vi "Data_Acquisition_10 sensors.vi"() -> ()   [LabVIEW 2020]
uses:
  <vilib>/Instr/_visa.llb/VISA Configure Serial Port (Instr).vi
panel:
  out "Path S10":path
  out "Path S9":path
  out "Path S8":path
  out "Path S7":path
  out "Path S6":path
  out "Path S5":path
  out "Path S3":path
  out "Path S4":path
  out "Path S2":path
  out "Path S1":path
  in  "Trial Select":string(combo)
  in  "Person Select":string(combo)
  in  "Gesture Select":string(combo)
  out "Myoware 2":dbl[](array[numeric]) format="%#.11g"
  out "FSR 8":dbl[](array[numeric]) format="%#.11g"
  out "FSR 7":dbl[](array[numeric]) format="%#.11g"
  out "FSR 6":dbl[](array[numeric]) format="%#.11g"
  out "FSR 5":dbl[](array[numeric]) format="%#.11g"
  out "Myoware 1":dbl[](array[numeric]) format="%#.11g"
  out "FSR 4":dbl[](array[numeric]) format="%#.11g"
  out "FSR 3":dbl[](array[numeric]) format="%#.11g"
  out "Myoware 2 Chart":dbl[](graph)
  out "FSR 8 Chart":dbl[](graph)
  out "FSR 7 Chart":dbl[](graph)
  out "FSR 6 Chart":dbl[](graph)
  out "FSR 5 Chart":dbl[](graph)
  out "Myoware 1 Chart":dbl[](graph)
  out "FSR 4 Chart":dbl[](graph)
  out "FSR 3 Chart":dbl[](graph)
  out "FSR 2 Chart":dbl[](graph)
  out "FSR 1 Chart":dbl[](graph)
  out "FSR 2":dbl[](array[numeric]) format="%#.11g"
  out "FSR 1":dbl[](array[numeric]) format="%#.11g"
  in  "COM Port Select":refnum<visa-resource-name>
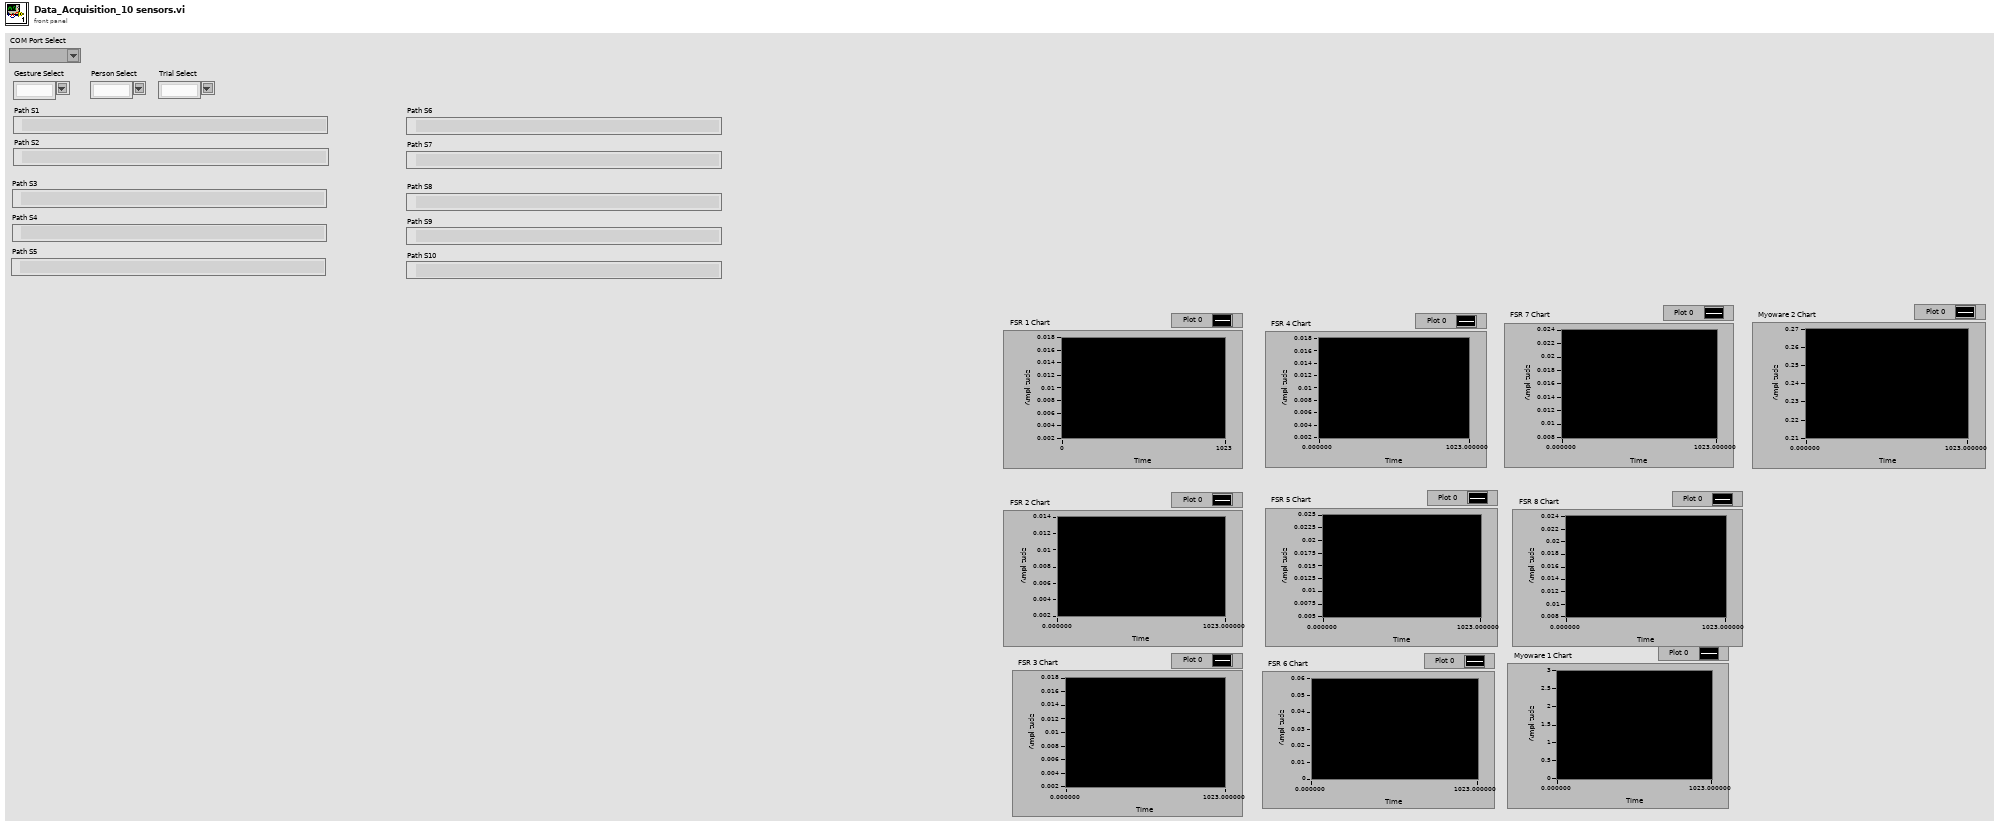
[diagram p1: front panel]
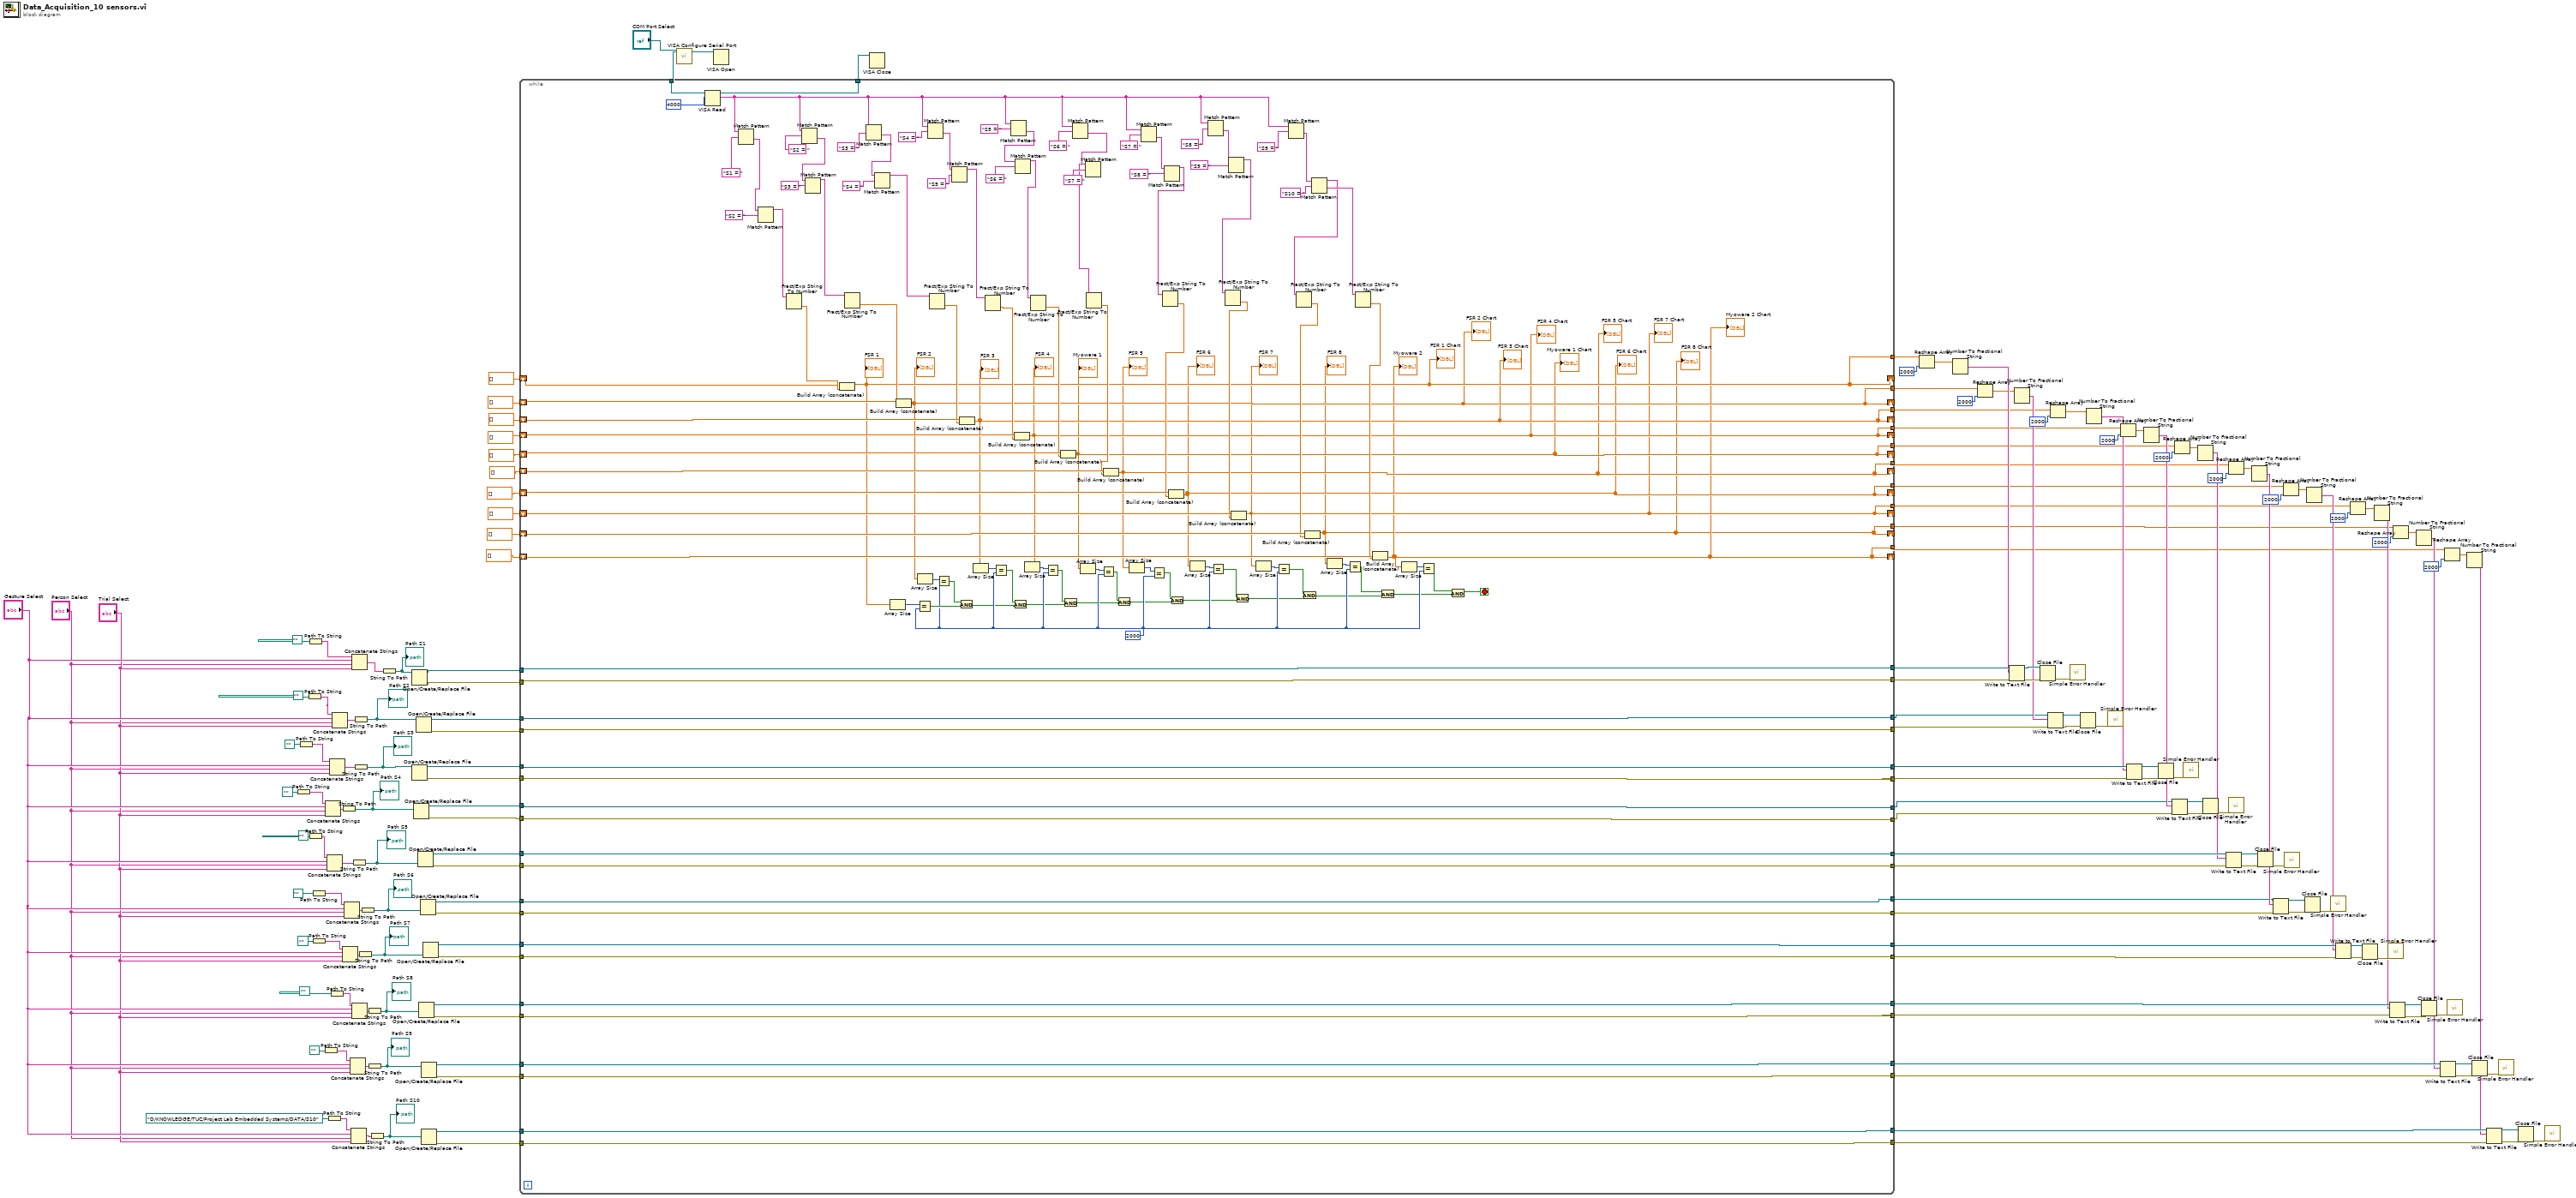
[diagram p0: block diagram]
diagram:
  n1 = Path To String(path=path "" ("file path (use dialog)")) -> (string=w142:string)
  n2 = Path To String(path=path "" ("file path (use dialog)")) -> (string=w139:string)
  n3 = Path To String(path=path "" ("file path (use dialog)")) -> (string=w146:string)
  n4 = Path To String(path=path "" ("file path (use dialog)")) -> (string=w152:string)
  n5 = Path To String(path=path "" ("file path (use dialog)")) -> (string=w136:string)
  n6 = Path To String(path=path "" ("file path (use dialog)")) -> (string=w130:string)
  n7 = Path To String(path=path "" ("file path (use dialog)")) -> (string=w133:string)
  n8 = Path To String(path=path "" ("file path (use dialog)")) -> (string=w124:string)
  n9 = Concatenate Strings(w142, "Gesture Select", "Person Select", "Trial Select") -> (w144:string)
  n10 = Path To String(path=path "D:/KNOWLEDGE/TUC/Project Lab Embedded Systems/DATA/S10" ("file path (use dialog)")) -> (string=w122:string)
  n11 = Concatenate Strings(w136, "Gesture Select", "Person Select", "Trial Select") -> (w138:string)
  n12 = Concatenate Strings(w139, "Gesture Select", "Person Select", "Trial Select") -> (w141:string)
  n13 = Path To String(path=path "" ("file path (use dialog)")) -> (string=w127:string)
  n14 = Concatenate Strings(w146, "Gesture Select", "Person Select", "Trial Select") -> (w145:string)
  n15 = String To Path(string=w144) -> (path=w96:path)
  "Path S4" <- w96
  n16 = Concatenate Strings(w130, "Gesture Select", "Person Select", "Trial Select") -> (w132:string)
  n17 = Concatenate Strings(w133, "Gesture Select", "Person Select", "Trial Select") -> (w135:string)
  n18 = Concatenate Strings(w124, "Gesture Select", "Person Select", "Trial Select") -> (w126:string)
  n19 = Concatenate Strings(w122, "Gesture Select", "Person Select", "Trial Select") -> (w123:string)
  n20 = Concatenate Strings(w152, "Gesture Select", "Person Select", "Trial Select") -> (w151:string)
  n21 = String To Path(string=w138) -> (path=w99:path)
  "Path S5" <- w99
  n22 = Concatenate Strings(w127, "Gesture Select", "Person Select", "Trial Select") -> (w129:string)
  n23 = String To Path(string=w145) -> (path=w91:path)
  "Path S2" <- w91
  n24 = String To Path(string=w141) -> (path=w97:path)
  "Path S3" <- w97
  n25 = String To Path(string=w132) -> (path=w92:path)
  "Path S7" <- w92
  n26 = String To Path(string=w135) -> (path=w98:path)
  "Path S6" <- w98
  n27 = String To Path(string=w126) -> (path=w94:path)
  "Path S9" <- w94
  n28 = String To Path(string=w129) -> (path=w93:path)
  "Path S8" <- w93
  n29 = String To Path(string=w123) -> (path=w95:path)
  "Path S10" <- w95
  n30 = String To Path(string=w151) -> (path=w148:path)
  "Path S1" <- w148
  n31 = Open/Create/Replace File(file path (use dialog)=w148) -> (refnum out=w150:refnum<file>, error out=w149:errorcluster)  [unwired: 5 in, 1 out]
  n32 = Open/Create/Replace File(file path (use dialog)=w97) -> (refnum out=w115:refnum<file>, error out=w114:errorcluster)  [unwired: 5 in, 1 out]
  n33 = Open/Create/Replace File(file path (use dialog)=w96) -> (refnum out=w113:refnum<file>, error out=w112:errorcluster)  [unwired: 5 in, 1 out]
  n34 = Open/Create/Replace File(file path (use dialog)=w91) -> (refnum out=w117:refnum<file>, error out=w116:errorcluster)  [unwired: 5 in, 1 out]
  n35 = Open/Create/Replace File(file path (use dialog)=w99) -> (refnum out=w111:refnum<file>, error out=w110:errorcluster)  [unwired: 5 in, 1 out]
  n36 = Open/Create/Replace File(file path (use dialog)=w93) -> (refnum out=w104:refnum<file>, error out=w105:errorcluster)  [unwired: 5 in, 1 out]
  n37 = Open/Create/Replace File(file path (use dialog)=w98) -> (refnum out=w108:refnum<file>, error out=w109:errorcluster)  [unwired: 5 in, 1 out]
  n38 = Open/Create/Replace File(file path (use dialog)=w94) -> (refnum out=w102:refnum<file>, error out=w103:errorcluster)  [unwired: 5 in, 1 out]
  n39 = Open/Create/Replace File(file path (use dialog)=w95) -> (refnum out=w100:refnum<file>, error out=w101:errorcluster)  [unwired: 5 in, 1 out]
  n40 = Open/Create/Replace File(file path (use dialog)=w92) -> (refnum out=w106:refnum<file>, error out=w107:errorcluster)  [unwired: 5 in, 1 out]
  n41 = call-poly "VISA Configure Serial Port"("VISA resource name"="COM Port Select") -> ("VISA resource name out"=w166:refnum<visa-resource-name>)  [unwired: 13 in, 1 out]
  n42 = VISA Open(VISA resource name=w166) -> (VISA resource name=w155:refnum<visa-resource-name>)  [unwired: 4 in, 1 out]
  n43 = while {
    shift-right: [w195] -> _
    shift-left: dbl[] [] -> [w288]
    shift-right: [w198] -> _
    shift-left: dbl[] [] -> [w199]
    shift-right: [w192] -> _
    shift-left: dbl[] [] -> [w283]
    shift-right: [w189] -> _
    shift-left: dbl[] [] -> [w279]
    shift-right: [w186] -> _
    shift-left: dbl[] [] -> [w278]
    shift-right: [w185] -> _
    shift-left: dbl[] [] -> [w282]
    shift-right: [w184] -> _
    shift-left: dbl[] [] -> [w277]
    shift-right: [w183] -> _
    shift-left: dbl[] [] -> [w281]
    shift-right: [w174] -> _
    shift-left: dbl[] [] -> [w280]
    shift-right: [w182] -> _
    shift-left: dbl[] [] -> [w276]
    tunnel: w155 -> [w239]
    tunnel: [w229] -> w154
    tunnel: w150 -> [w197]
    tunnel: w149 -> [w196]
    tunnel: w117 -> [w194]
    tunnel: w116 -> [w193]
    tunnel: [w193] -> w73
    tunnel: [w194] -> w74
    tunnel: w115 -> [w191]
    tunnel: w114 -> [w190]
    tunnel: w113 -> [w188]
    tunnel: w112 -> [w187]
    tunnel: w111 -> [w171]
    tunnel: w110 -> [w170]
    tunnel: w109 -> [w172]
    tunnel: w108 -> [w173]
    tunnel: w107 -> [w175]
    tunnel: w106 -> [w169]
    tunnel: w105 -> [w177]
    tunnel: w104 -> [w176]
    tunnel: w103 -> [w179]
    tunnel: w102 -> [w178]
    tunnel: w101 -> [w181]
    tunnel: w100 -> [w180]
    tunnel: [w191] -> w68
    tunnel: [w190] -> w67
    tunnel: [w188] -> w56
    tunnel: [w187] -> w55
    tunnel: [w171] -> w51
    tunnel: [w170] -> w50
    tunnel: [w173] -> w38
    tunnel: [w172] -> w37
    tunnel: [w169] -> w33
    tunnel: [w175] -> w32
    tunnel: [w176] -> w28
    tunnel: [w177] -> w27
    tunnel: [w178] -> w23
    tunnel: [w179] -> w22
    tunnel: [w180] -> w18
    tunnel: [w181] -> w17
    tunnel: [w198] -> w89
    tunnel: [w197] -> w84
    tunnel: [w196] -> w83
    tunnel: [w195] -> w76
    tunnel: [w192] -> w70
    tunnel: [w189] -> w61
    tunnel: [w186] -> w47
    tunnel: [w185] -> w43
    tunnel: [w184] -> w14
    tunnel: [w183] -> w10
    tunnel: [w174] -> w6
    tunnel: [w182] -> w2
    stop <- w168 stop-if-true
    w267 = 2000 ("y")
    n44 = VISA Read(VISA resource name=w239, byte count=u32 4000) -> (VISA resource name out=w229:refnum<visa-resource-name>, read buffer=w204:string)  [unwired: 1 in, 2 out]
    n45 = Match Pattern(string=w204, regular expression="S1 = ") -> (after substring=w225:string)  [unwired: 1 in, 3 out]
    n46 = Match Pattern(string=w225, regular expression="S2 = ") -> (before substring=w226:string)  [unwired: 1 in, 3 out]
    n47 = Fract/Exp String To Number(string=w226) -> (number=w230:dbl)  [unwired: 3 in, 1 out]
    n48 = Match Pattern(string=w204, regular expression="S2 = ") -> (after substring=w223:string)  [unwired: 1 in, 3 out]
    n49 = Match Pattern(string=w223, regular expression="S3 = ") -> (before substring=w222:string)  [unwired: 1 in, 3 out]
    n50 = Build Array (concatenate)(w199, w230) -> (w198:dbl[])
    "FSR 1" <- w198
    "FSR 1 Chart" <- w198
    n51 = Fract/Exp String To Number(string=w222) -> (number=w231:dbl)  [unwired: 3 in, 1 out]
    n52 = Match Pattern(string=w204, regular expression="S3 = ") -> (after substring=w220:string)  [unwired: 1 in, 3 out]
    n53 = Match Pattern(string=w220, regular expression="S4 = ") -> (before substring=w219:string)  [unwired: 1 in, 3 out]
    n54 = Array Size(array=w198) -> (size(s)=w286:i32)
    n55 = Build Array (concatenate)(w288, w231) -> (w195:dbl[])
    "FSR 2" <- w195
    "FSR 2 Chart" <- w195
    n56 = Array Size(array=w195) -> (size(s)=w287:i32)
    n57 = Equal?(x=w286, y=w267) -> (x = y?=w284:bool)
    n58 = Match Pattern(string=w204, regular expression="S4 = ") -> (after substring=w217:string)  [unwired: 1 in, 3 out]
    n59 = Fract/Exp String To Number(string=w219) -> (number=w232:dbl)  [unwired: 3 in, 1 out]
    n60 = Equal?(x=w287, y=w267) -> (x = y?=w285:bool)
    n61 = Match Pattern(string=w217, regular expression="S5 = ") -> (before substring=w216:string)  [unwired: 1 in, 3 out]
    n62 = And(x=w285, y=w284) -> (x .and. y?=w265:bool)
    n63 = Build Array (concatenate)(w283, w232) -> (w192:dbl[])
    "FSR 3 Chart" <- w192
    "FSR 3" <- w192
    n64 = Array Size(array=w192) -> (size(s)=w275:i32)
    n65 = Fract/Exp String To Number(string=w216) -> (number=w233:dbl)  [unwired: 3 in, 1 out]
    n66 = Equal?(x=w275, y=w267) -> (x = y?=w266:bool)
    n67 = Match Pattern(string=w204, regular expression="S5 = ") -> (after substring=w214:string)  [unwired: 1 in, 3 out]
    n68 = And(x=w266, y=w265) -> (x .and. y?=w264:bool)
    n69 = Build Array (concatenate)(w279, w233) -> (w189:dbl[])
    "FSR 4 Chart" <- w189
    "FSR 4" <- w189
    n70 = Match Pattern(string=w214, regular expression="S6 = ") -> (before substring=w213:string)  [unwired: 1 in, 3 out]
    n71 = Array Size(array=w189) -> (size(s)=w274:i32)
    n72 = Fract/Exp String To Number(string=w213) -> (number=w234:dbl)  [unwired: 3 in, 1 out]
    n73 = Equal?(x=w274, y=w267) -> (x = y?=w263:bool)
    n74 = Build Array (concatenate)(w278, w234) -> (w186:dbl[])
    "Myoware 1 Chart" <- w186
    "Myoware 1" <- w186
    n75 = And(x=w263, y=w264) -> (x .and. y?=w262:bool)
    n76 = Match Pattern(string=w204, regular expression="S6 = ") -> (after substring=w211:string)  [unwired: 1 in, 3 out]
    n77 = Array Size(array=w186) -> (size(s)=w273:i32)
    n78 = Match Pattern(string=w211, regular expression="S7 = ") -> (before substring=w210:string)  [unwired: 1 in, 3 out]
    n79 = Fract/Exp String To Number(string=w210) -> (number=w235:dbl)  [unwired: 3 in, 1 out]
    n80 = Equal?(x=w273, y=w267) -> (x = y?=w261:bool)
    n81 = Build Array (concatenate)(w282, w235) -> (w185:dbl[])
    "FSR 5 Chart" <- w185
    "FSR 5" <- w185
    n82 = And(x=w261, y=w262) -> (x .and. y?=w260:bool)
    n83 = Array Size(array=w185) -> (size(s)=w272:i32)
    n84 = Match Pattern(string=w204, regular expression="S7 = ") -> (after substring=w200:string)  [unwired: 1 in, 3 out]
    n85 = Equal?(x=w272, y=w267) -> (x = y?=w259:bool)
    n86 = Match Pattern(string=w200, regular expression="S8 = ") -> (before substring=w208:string)  [unwired: 1 in, 3 out]
    n87 = Fract/Exp String To Number(string=w208) -> (number=w236:dbl)  [unwired: 3 in, 1 out]
    n88 = Build Array (concatenate)(w277, w236) -> (w184:dbl[])
    "FSR 6 Chart" <- w184
    "FSR 6" <- w184
    n89 = And(x=w259, y=w260) -> (x .and. y?=w258:bool)
    n90 = Array Size(array=w184) -> (size(s)=w271:i32)
    n91 = Match Pattern(string=w204, regular expression="S8 = ") -> (after substring=w206:string)  [unwired: 1 in, 3 out]
    n92 = Equal?(x=w271, y=w267) -> (x = y?=w257:bool)
    n93 = Match Pattern(string=w206, regular expression="S9 = ") -> (before substring=w205:string)  [unwired: 1 in, 3 out]
    n94 = Fract/Exp String To Number(string=w205) -> (number=w237:dbl)  [unwired: 3 in, 1 out]
    n95 = Build Array (concatenate)(w281, w237) -> (w183:dbl[])
    "FSR 7 Chart" <- w183
    "FSR 7" <- w183
    n96 = And(x=w257, y=w258) -> (x .and. y?=w256:bool)
    n97 = Array Size(array=w183) -> (size(s)=w270:i32)
    n98 = Equal?(x=w270, y=w267) -> (x = y?=w255:bool)
    n99 = Match Pattern(string=w204, regular expression="S9 = ") -> (after substring=w202:string)  [unwired: 1 in, 3 out]
    n100 = And(x=w255, y=w256) -> (x .and. y?=w254:bool)
    n101 = Match Pattern(string=w202, regular expression="S10 = ") -> (before substring=w249:string, after substring=w250:string)  [unwired: 1 in, 2 out]
    n102 = Fract/Exp String To Number(string=w249) -> (number=w238:dbl)  [unwired: 3 in, 1 out]
    n103 = Build Array (concatenate)(w280, w238) -> (w174:dbl[])
    "FSR 8 Chart" <- w174
    "FSR 8" <- w174
    n104 = Array Size(array=w174) -> (size(s)=w269:i32)
    n105 = Equal?(x=w269, y=w267) -> (x = y?=w253:bool)
    n106 = Fract/Exp String To Number(string=w250) -> (number=w201:dbl)  [unwired: 3 in, 1 out]
    n107 = Build Array (concatenate)(w276, w201) -> (w182:dbl[])
    "Myoware 2 Chart" <- w182
    "Myoware 2" <- w182
    n108 = And(x=w253, y=w254) -> (x .and. y?=w252:bool)
    n109 = Array Size(array=w182) -> (size(s)=w268:i32)
    n110 = Equal?(x=w268, y=w267) -> (x = y?=w251:bool)
    n111 = And(x=w251, y=w252) -> (x .and. y?=w168:bool)
  }
  n112 = VISA Close(VISA resource name=w154) -> ()  [unwired: 1 in, 1 out]
  n113 = Reshape Array(w89, 2000 ("dimension size")) -> (w88:dbl[])
  n114 = Number To Fractional String(number=w88) -> (F-format string=w82:string[])  [unwired: 3 in]
  n115 = Reshape Array(w76, 2000 ("dimension size")) -> (w77:dbl[])
  n116 = Write to Text File(file (use dialog)=w84, text=w82, error in=w83) -> (refnum out=w86:refnum<file>, error out=w85:errorcluster)  [unwired: 1 in, 1 out]
  n117 = Number To Fractional String(number=w77) -> (F-format string=w75:string[])  [unwired: 3 in]
  n118 = Close File(refnum=w86, error in=w85) -> (error out=w87:errorcluster)  [unwired: 1 out]
  n119 = Write to Text File(file (use dialog)=w74, text=w75, error in=w73) -> (refnum out=w80:refnum<file>, error out=w79:errorcluster)  [unwired: 1 in, 1 out]
  n120 = Reshape Array(w70, 2000 ("dimension size")) -> (w71:dbl[])
  n121 = call <vilib>:"Simple Error Handler.vi"("error in (no error)"=w87) -> ()  [unwired: 4 in, 5 out]
  n122 = Close File(refnum=w80, error in=w79) -> (error out=w81:errorcluster)  [unwired: 1 out]
  n123 = Number To Fractional String(number=w71) -> (F-format string=w64:string[])  [unwired: 3 in]
  n124 = call <vilib>:"Simple Error Handler.vi"("error in (no error)"=w81) -> ()  [unwired: 4 in, 5 out]
  n125 = Reshape Array(w61, 2000 ("dimension size")) -> (w62:dbl[])
  n126 = Write to Text File(file (use dialog)=w68, text=w64, error in=w67) -> (refnum out=w66:refnum<file>, error out=w65:errorcluster)  [unwired: 1 in, 1 out]
  n127 = Number To Fractional String(number=w62) -> (F-format string=w57:string[])  [unwired: 3 in]
  n128 = Close File(refnum=w66, error in=w65) -> (error out=w69:errorcluster)  [unwired: 1 out]
  n129 = Write to Text File(file (use dialog)=w56, text=w57, error in=w55) -> (refnum out=w59:refnum<file>, error out=w58:errorcluster)  [unwired: 1 in, 1 out]
  n130 = Reshape Array(w47, 2000 ("dimension size")) -> (w48:dbl[])
  n131 = call <vilib>:"Simple Error Handler.vi"("error in (no error)"=w69) -> ()  [unwired: 4 in, 5 out]
  n132 = Number To Fractional String(number=w48) -> (F-format string=w46:string[])  [unwired: 3 in]
  n133 = Close File(refnum=w59, error in=w58) -> (error out=w60:errorcluster)  [unwired: 1 out]
  n134 = Write to Text File(file (use dialog)=w51, text=w46, error in=w50) -> (refnum out=w53:refnum<file>, error out=w52:errorcluster)  [unwired: 1 in, 1 out]
  n135 = Reshape Array(w43, 2000 ("dimension size")) -> (w44:dbl[])
  n136 = call <vilib>:"Simple Error Handler.vi"("error in (no error)"=w60) -> ()  [unwired: 4 in, 5 out]
  n137 = Number To Fractional String(number=w44) -> (F-format string=w39:string[])  [unwired: 3 in]
  n138 = Close File(refnum=w53, error in=w52) -> (error out=w54:errorcluster)  [unwired: 1 out]
  n139 = Write to Text File(file (use dialog)=w38, text=w39, error in=w37) -> (refnum out=w41:refnum<file>, error out=w40:errorcluster)  [unwired: 1 in, 1 out]
  n140 = Reshape Array(w14, 2000 ("dimension size")) -> (w15:dbl[])
  n141 = call <vilib>:"Simple Error Handler.vi"("error in (no error)"=w54) -> ()  [unwired: 4 in, 5 out]
  n142 = Close File(refnum=w41, error in=w40) -> (error out=w42:errorcluster)  [unwired: 1 out]
  n143 = Number To Fractional String(number=w15) -> (F-format string=w13:string[])  [unwired: 3 in]
  n144 = call <vilib>:"Simple Error Handler.vi"("error in (no error)"=w42) -> ()  [unwired: 4 in, 5 out]
  n145 = Write to Text File(file (use dialog)=w33, text=w13, error in=w32) -> (refnum out=w35:refnum<file>, error out=w34:errorcluster)  [unwired: 1 in, 1 out]
  n146 = Reshape Array(w10, 2000 ("dimension size")) -> (w11:dbl[])
  n147 = Close File(refnum=w35, error in=w34) -> (error out=w36:errorcluster)  [unwired: 1 out]
  n148 = Number To Fractional String(number=w11) -> (F-format string=w9:string[])  [unwired: 3 in]
  n149 = call <vilib>:"Simple Error Handler.vi"("error in (no error)"=w36) -> ()  [unwired: 4 in, 5 out]
  n150 = Write to Text File(file (use dialog)=w28, text=w9, error in=w27) -> (refnum out=w30:refnum<file>, error out=w29:errorcluster)  [unwired: 1 in, 1 out]
  n151 = Reshape Array(w6, 2000 ("dimension size")) -> (w7:dbl[])
  n152 = Number To Fractional String(number=w7) -> (F-format string=w5:string[])  [unwired: 3 in]
  n153 = Close File(refnum=w30, error in=w29) -> (error out=w31:errorcluster)  [unwired: 1 out]
  n154 = Write to Text File(file (use dialog)=w23, text=w5, error in=w22) -> (refnum out=w25:refnum<file>, error out=w24:errorcluster)  [unwired: 1 in, 1 out]
  n155 = Reshape Array(w2, 2000 ("dimension size")) -> (w3:dbl[])
  n156 = call <vilib>:"Simple Error Handler.vi"("error in (no error)"=w31) -> ()  [unwired: 4 in, 5 out]
  n157 = Number To Fractional String(number=w3) -> (F-format string=w1:string[])  [unwired: 3 in]
  n158 = Close File(refnum=w25, error in=w24) -> (error out=w26:errorcluster)  [unwired: 1 out]
  n159 = Write to Text File(file (use dialog)=w18, text=w1, error in=w17) -> (refnum out=w20:refnum<file>, error out=w19:errorcluster)  [unwired: 1 in, 1 out]
  n160 = call <vilib>:"Simple Error Handler.vi"("error in (no error)"=w26) -> ()  [unwired: 4 in, 5 out]
  n161 = Close File(refnum=w20, error in=w19) -> (error out=w21:errorcluster)  [unwired: 1 out]
  n162 = call <vilib>:"Simple Error Handler.vi"("error in (no error)"=w21) -> ()  [unwired: 4 in, 5 out]
